vi "Generate Unique Server ID.vi"(8 "error in (no error)":errorcluster, 10 "Variant":variant, 11 "server id in":i32) -> (0 "error out":errorcluster, 3 "unique server id out":i32)   [LabVIEW 2020, in "MCP Server.lvlib"]
doc: "Generates a unique id for the server. Increments if the id already exists. Timeouts after 10k ids."
uses:
  MCP Server.lvlib
  <vilib>/Utility/error.llb/Error Cluster From Error Code.vi
  <vilib>/ErrorRing/Error Ring.xnode
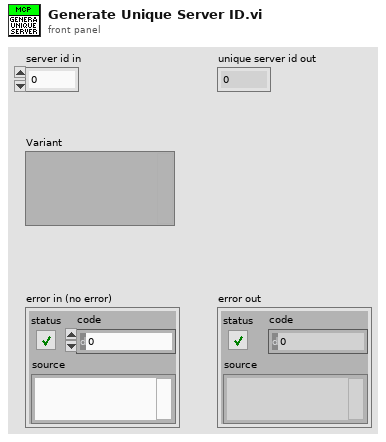
[diagram p1: front panel]
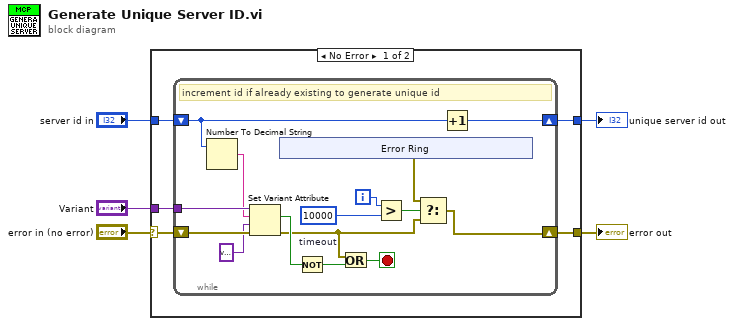
[diagram p0: block diagram]
diagram:
  n1 = case shown="No Error" "error in (no error)" {
    selector: "error in (no error)" -> [w6 w31]
    tunnel: [w10 w32] -> w5
    tunnel: "server id in" -> [w9 w32]
    tunnel: [w8 w31] -> w3
    tunnel: "Variant" -> [w7 _]
    frame No Error {
      n2 = while {
        tunnel: w7 -> [w25]
        shift-right: [w14] -> w8
        shift-left: w6 -> [w24]
        shift-right: [w17] -> w10
        shift-left: w9 -> [w18]
        i -> [w16]
        stop <- w21 stop-if-true
        w15 = 10000  # timeout
        # "increment id if already existing to generate unique id"
        n3 = Number To Decimal String(number=w18) -> (decimal integer string=w19:string)  [unwired: 1 in]
        n4 = Set Variant Attribute(Variant=w25, name=w19, value=variant, error in=w24) -> (replaced=w23:bool, error out=w20:errorcluster)  [unwired: 1 out]
        n5 = xnode "Error Ring"() -> ("error out"=w12:errorcluster)
        n6 = Not(x=w23) -> (.not. x?=w22:bool)
        n7 = Or(x=w20, y=w22) -> (x .or. y?=w21:bool)
        n8 = Greater?(x=w16, y=w15) -> (0:w13:bool)
        n9 = Select(t=w12, s=w13, f=w20) -> (s? t:f=w14:errorcluster)
        n10 = Increment(x=w18) -> (x+1=w17:i32)
      }
    }
    frame Error {
    }
  }
  "unique server id out" <- w5
  "error out" <- w3
